vi "BACKUP_Keithley2450_and_24xx_plus_lockin_7_14_24.vi"() -> ()   [LabVIEW 2024]
uses:
  <vilib>/Analysis/1siggen.llb/Ramp Pattern by Delta.vi
  <vilib>/Utility/file.llb/Write Delimited Spreadsheet (string).vi
  <vilib>/Utility/file.llb/Write Delimited Spreadsheet (DBL).vi
  C:/Users/Public/OneDrive/Desktop/Keithley_2450_2470_1_4_0_LV2015_NewReadme2_2450-LV2015-1.4.0/Keithley 2450/Keithley 2450.lvlib
  <vilib>/Analysis/NI_AALBase.lvlib
  archive/Keithley 24XX/Keithley 24XX.lvlib
panel:
  out "XY Graph 3":cluster{dbl[], dbl[]}(graph)={[0.0, 0.05, 0.1, 0.15000000000000002, 0.2, 0.25, 0.30000000000000004, 0.35000000000000003, 0.4], [2.058748289029846, 2.0549935802361086, 2.025945473215966, 1.958083977655374, 1.8694392276726999, 1.770704656221769, 1.6639789912388152, 1.559635375168859, 1.4675568762085736]}
  out "current E field":dbl=0.4
  in  "d_t":dbl=17.0 format="%#_13g"
  in  "d_b":dbl=17.0 format="%#_13g"
  in  "E step":dbl=0.05 format="%#_13g"
  in  "E end":dbl=0.4 format="%#_13g"
  in  "E start (v/nm)":dbl format="%#_13g"
  out "current voltage 2450":dbl=6.7979141 format="%0.4f"
  in  "Reverse 2410":bool
  in  "Serial Configuration 2":T1={"Baud Rate"=9600, "Parity"=0, "Data Bits"=8, "Stop Bits"=10, "Flow Control"=0} {"Flow Control" items=["None", "XON/XOFF", "RTS/CTS", "XON/XOFF & RTS/CTS", "DTR/DSR", "XON/XOFF & DTR/DSR"]; "Stop Bits" items=["1.0"=10, "1.5"=15, "2.0"=20]; "Data Bits" items=["7"=7, "8"=8]; "Parity" items=["None", "Odd", "Even", "Mark", "Space"]; "Baud Rate" items=["300"=300, "600"=600, "1200"=1200, "2400"=2400, "4800"=4800, "9600"=9600, "19200"=19200]}
  in  "reset":bool
  in  "use 2540?":bool=TRUE
  out "XY Graph 2":cluster{dbl[], dbl[]}(graph)={[0.0, 0.05, 0.1, 0.15000000000000002, 0.2, 0.25, 0.30000000000000004, 0.35000000000000003, 0.4], [-0.0003388190682879211, 0.0003901722529266183, 1.3430241380812946e-05, 1.333691247717983e-05, 0.0001438023883998385, -0.0008806402301830829, -0.0010907914765878601, -0.0006143232866850923, -0.0016053824714035159]}
  out "XY Graph":cluster{dbl[], dbl[]}(graph)={[0.0, 0.05, 0.1, 0.15000000000000002, 0.2, 0.25, 0.30000000000000004, 0.35000000000000003, 0.4], [2.058748289029846, 2.0549935802361086, 2.025945473215966, 1.958083977655374, 1.8694392276726999, 1.770704656221769, 1.6639789912388152, 1.559635375168859, 1.4675568762085736]}
  in  "using 2400?":bool=TRUE
  out "current voltage 2410":dbl=-6.799285054206848 format="%0.4f"
  out "Current set voltage 2410":dbl=-6.800000000000001
  in  "V stepsize 2410":dbl
  in  "start V 2410":dbl
  in  "End V 2410":dbl
  out "standard deviation current measured 2450":dbl=1.0038305493714546e-08 format="%0.5e"
  out "mean current measured 2450":dbl=1.7421272433999997e-09 format="%0.5e"
  out "standard deviation current measured 2410":dbl=4.5644384533816545e-09 format="%0.5e"
  out "mean current measured 2410":dbl=-1.605382471403516e-09 format="%0.5e"
  in  "Compliance  Level 2410":dbl=5e-08
  in  "VISA resource name 2410":refnum<visa-resource-name>="GPIB0::16::INSTR"
  in  "Serial Configuration":T1={"Baud Rate"=9600, "Parity"=0, "Data Bits"=8, "Stop Bits"=10, "Flow Control"=0} {"Flow Control" items=["None", "XON/XOFF", "RTS/CTS", "XON/XOFF & RTS/CTS", "DTR/DSR", "XON/XOFF & DTR/DSR"]; "Stop Bits" items=["1.0"=10, "1.5"=15, "2.0"=20]; "Data Bits" items=["7"=7, "8"=8]; "Parity" items=["None", "Odd", "Even", "Mark", "Space"]; "Baud Rate" items=["300"=300, "600"=600, "1200"=1200, "2400"=2400, "4800"=4800, "9600"=9600, "19200"=19200]}
  in  "Wait for Current Meas":u32=100
  in  "Number of Current Meas":u32=20
  in  "Loop?":bool
  out "Current set voltage 2450":dbl=6.800000000000001
  in  "V stepsize 2450":dbl=0.5
  in  "start V 2450":dbl
  in  "End V 2450":dbl=2.0
  in  "Wait for lock in meas (ms)":i32=1000
  in  "File Path":path=path "C:/Users/Public/OneDrive/Desktop/test.txt"
  out "错误输出":errorcluster={"status"=FALSE, "code"=1073676294, "source"="VISA Read in OE1022D_Query_Data.vi->Keithley2450_and_24xx_plus_lockin_7_14_24.vi"}
  in  "Channel A Waveform Display":string(combo)="A-R"
  in  "Channel B Waveform Display":string(combo)="Channel_B_Rh1"
  out "AUX-ADC4 (V)":sgl format="%.3f"
  out "AUX-ADC3 (V)":sgl=0.0024414062 format="%.3f"
  out "AUX-ADC1 (V)":sgl format="%.3f"
  out "AUX-ADC2 (V)":sgl=0.0048828125 format="%.3f"
  out "R":sgl=0.0014845738 caption="R (Vrms)" format="%.3p"
  out "X":sgl=0.0014822832 caption="X (Vrms)" format="%.3p"
  out "Y":sgl=8.243722e-05 caption="Y (Vrms)" format="%.3p"
  out "θ (°)":sgl=3.183227 caption="θ (deg)" format="%.2f"
  out "频率 (Hz)":sgl=6040.048 caption="Freq (Hz)" format="%#.3f"
  out "噪声":sgl=1.6480133e-06 caption="Noise(Vrms)" format="%.3p"
  out "Rh1":sgl=9.916211e-05 caption="Rh1 (Vrms)" format="%.3p"
  out "θh1 (°)":sgl=90.1837 caption="θh1 (deg)" format="%.2f"
  out "Xh1":sgl=-3.1792828e-07 caption="Xh1 (Vrms)" format="%.3p"
  out "Yh1":sgl=9.91616e-05 caption="Yh1 (Vrms)" format="%.3p"
  out "X 2":sgl=4.511473e-07 caption="X (Vrms)" format="%.3p"
  out "Y 2":sgl=-4.716565e-07 caption="Y (Vrms)" format="%.3p"
  out "R 2":sgl=6.5268193e-07 caption="R (Vrms)" format="%.3p"
  out "θ (°) 2":sgl=-46.273182 caption="θ (deg)" format="%.2f"
  out "频率 (Hz) 2":sgl=50065.285 caption="Freq (Hz)" format="%#.3f"
  out "噪声 2":sgl=7.305374e-08 caption="Noise(Vrms)" format="%.3p"
  out "Xh1 2":sgl=1.594661e-05 caption="Xh1 (Vrms)" format="%.3p"
  out "Yh1 2":sgl=1.481611e-05 caption="Yh1 (Vrms)" format="%.3p"
  out "Rh1 2":sgl=2.1767211e-05 caption="Rh1 (Vrms)" format="%.3p"
  out "θh1 (°) 2":sgl=42.895382 caption="θh1 (deg)" format="%.2f"
  in  "A Sensitivity":u16(ring)=22 items=["1 nV/fA", "2 nV/fA", "5 nV/fA", "10 nV/fA", "20 nV/fA", "50 nV/fA", "100 nV/fA", "200 nV/fA", "500 nV/fA", "1 uV/pA", "2 uV/pA", "5 uV/pA", "10 uV/pA", "20 uV/pA", "50 uV/pA", "100 uV/pA", "200 uV/pA", "500 uV/pA", "1 mV/nA", "2 mV/nA", "5 mV/nA", "10 mV/nA", "20 mV/nA", "50 mV/nA", "100 mV/nA", "200 mV/nA", "500 mV/nA", "1 V/uA"]
  in  "B Sensitivity":u16(ring)=18 items=["1 nV/fA", "2 nV/fA", "5 nV/fA", "10 nV/fA", "20 nV/fA", "50 nV/fA", "100 nV/fA", "200 nV/fA", "500 nV/fA", "1 uV/pA", "2 uV/pA", "5 uV/pA", "10 uV/pA", "20 uV/pA", "50 uV/pA", "100 uV/pA", "200 uV/pA", "500 uV/pA", "1 mV/nA", "2 mV/nA", "5 mV/nA", "10 mV/nA", "20 mV/nA", "50 mV/nA", "100 mV/nA", "200 mV/nA", "500 mV/nA", "1 V/uA"]
  out "序列号":string="SSI LIA-OE1022D,SN:D6712164,Ver6.3200831"
  in  "Num Lock in Points":i32=100
  in  "OE1022D":refnum<visa-resource-name>="COM4"
  in  "Current Compliance Limit (0.1) 2450":dbl=5e-08
  in  "VISA resource name 2450":refnum<visa-resource-name>="GPIB0::1::INSTR"
  # "D:\\LabData\\XiaoWang_Group_data_2024on\\StackingTransitions\\CrI3\\dual_gate_round4\\d3\\RMCD\\Esweeps_0T_after_m2T\\stacked_location1_scan1.txt"
  # "C:\\Users\\Public\\OneDrive\\Desktop\\test.txt"
  # "instruments need to be reset before this runs. Run the sub vis that reset them. This has to be done because we do not reset in our program. That would turn off the output but we want to leave that on."
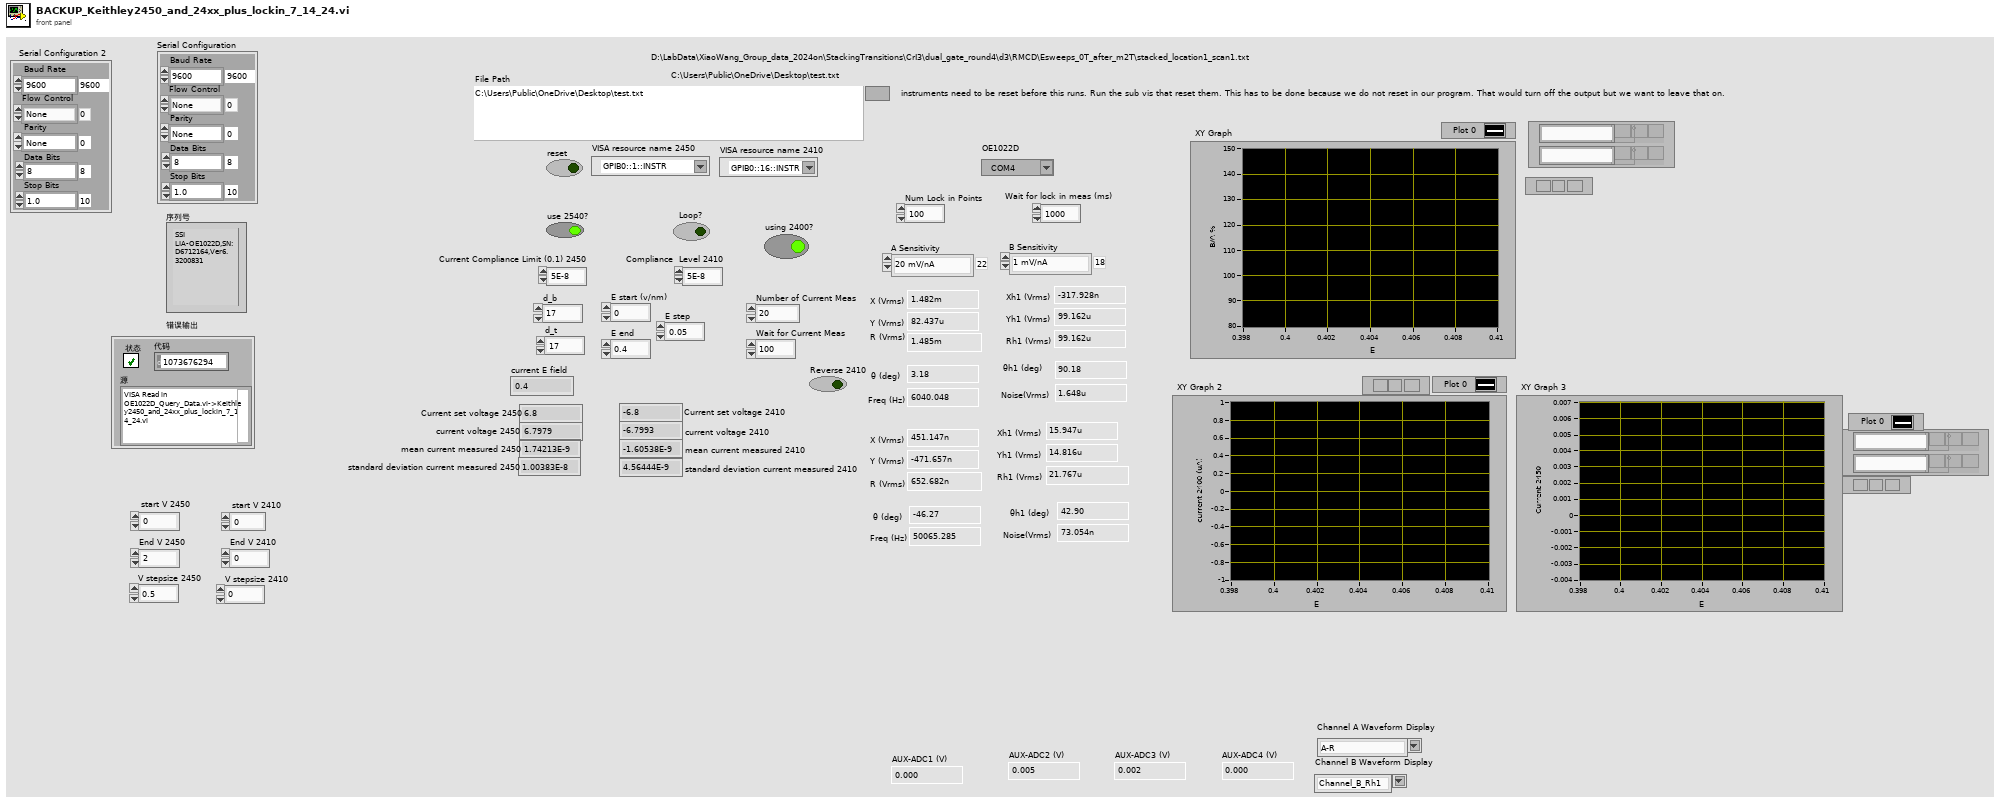
[diagram p1: front panel]
types:
  T1 = cluster{"Baud Rate":u32, "Parity":u16, "Data Bits":u16, "Stop Bits":u16, "Flow Control":u16}
  T2 = cluster{"AD1":dbl[], "AD2":dbl[], "AD3":dbl[], "AD4":dbl[]}
  T3 = cluster{"XB":dbl[], "YB":dbl[], "FrequencyB":dbl[], "NoiseB":dbl[], "Xh1B":dbl[], "Yh1B":dbl[], "Xh2B":dbl[], "Yh2B":dbl[], "Xh2B":dbl[]}
  T4 = cluster{"XA":dbl[], "YA":dbl[], "FrequencyA":dbl[], "NoiseA":dbl[], "Xh1A":dbl[], "Yh1A":dbl[], "Xh2A":dbl[], "Yh2A":dbl[]}
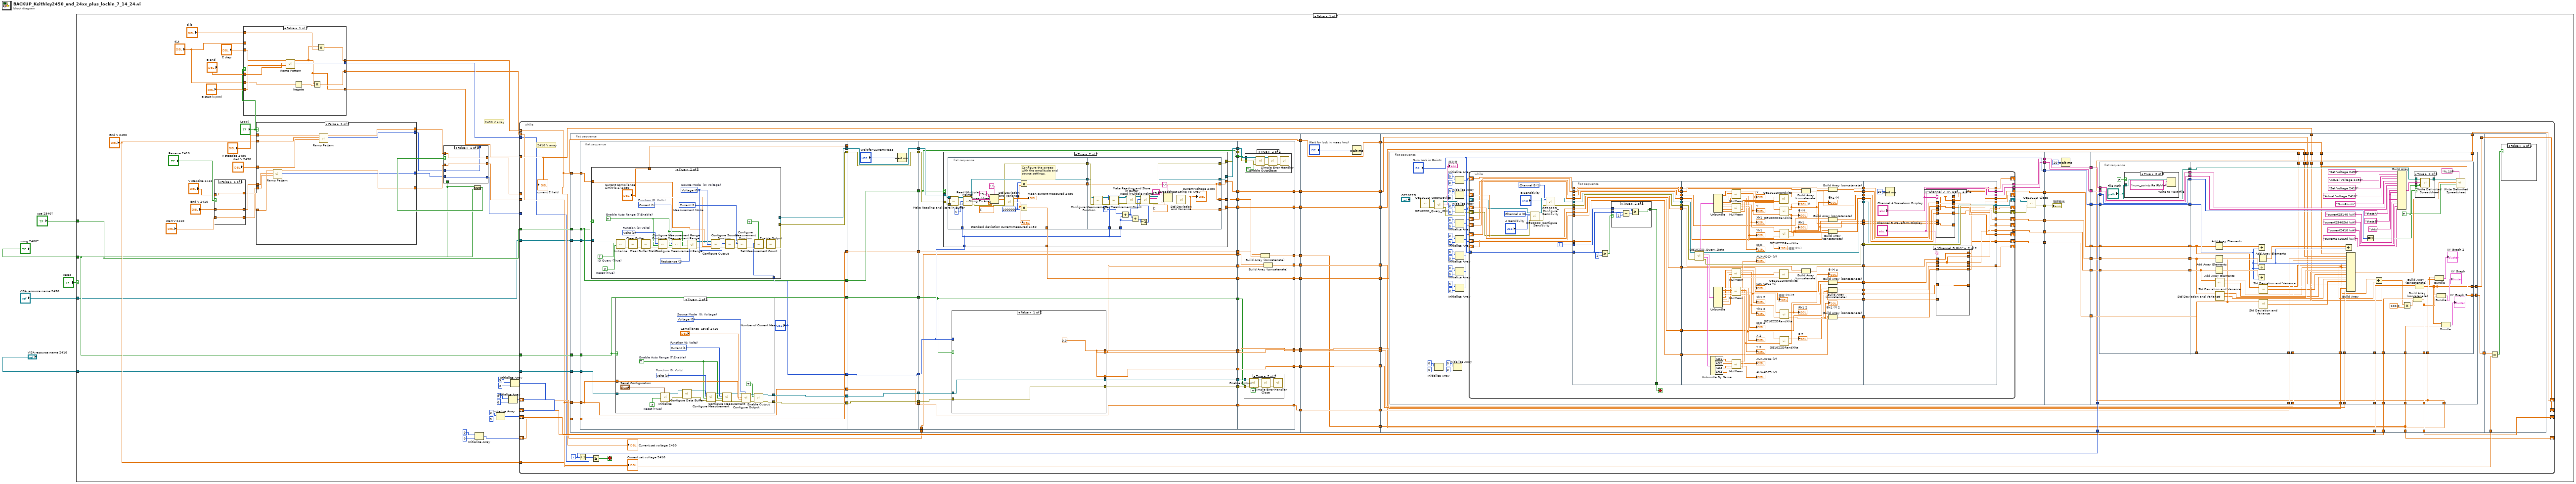
[diagram p0: block diagram]
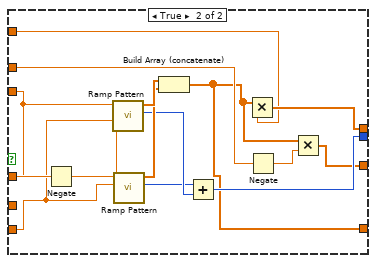
[diagram p2: hidden frame]
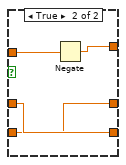
[diagram p3: hidden frame]
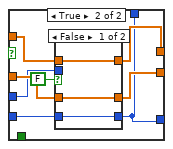
[diagram p4: hidden frame]
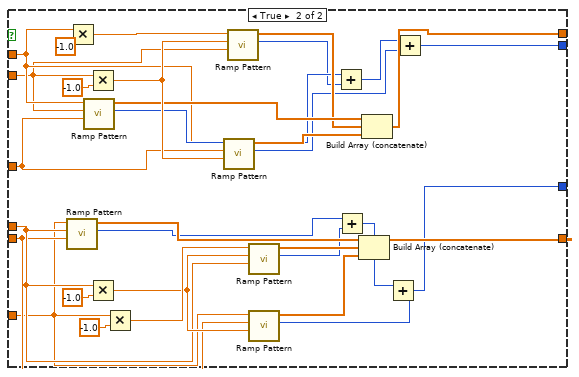
[diagram p6: hidden frame]
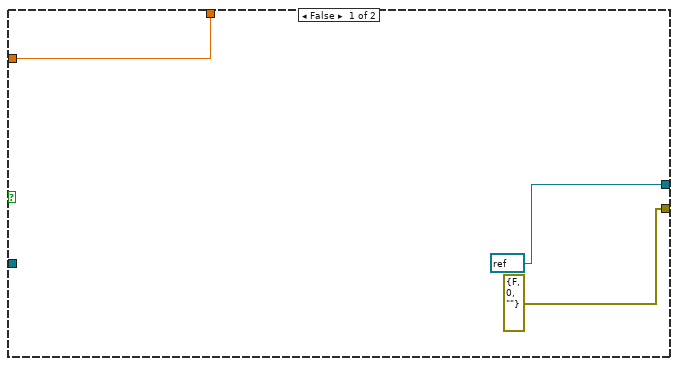
[diagram p7: hidden frame]
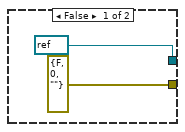
[diagram p8: hidden frame]
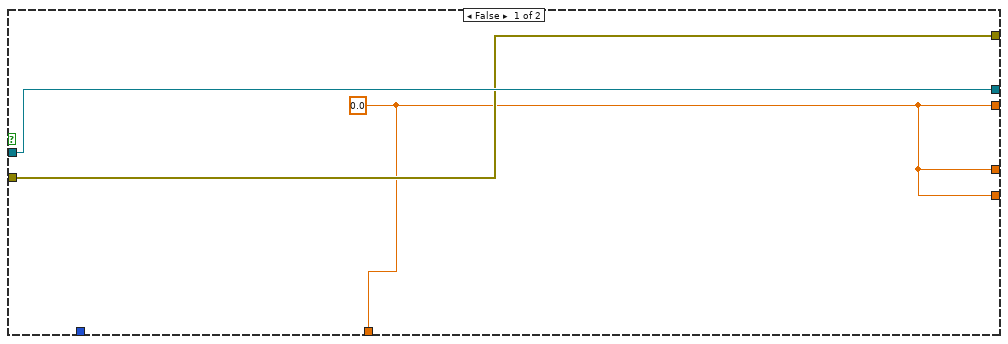
[diagram p9: hidden frame]
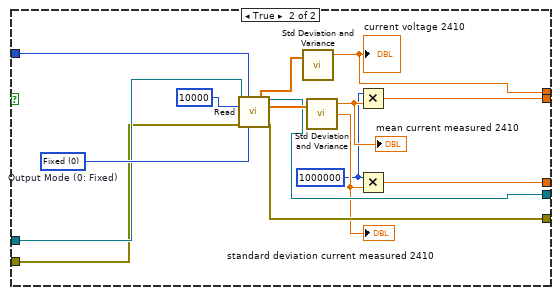
[diagram p10: hidden frame]
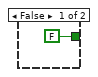
[diagram p13: hidden frame]
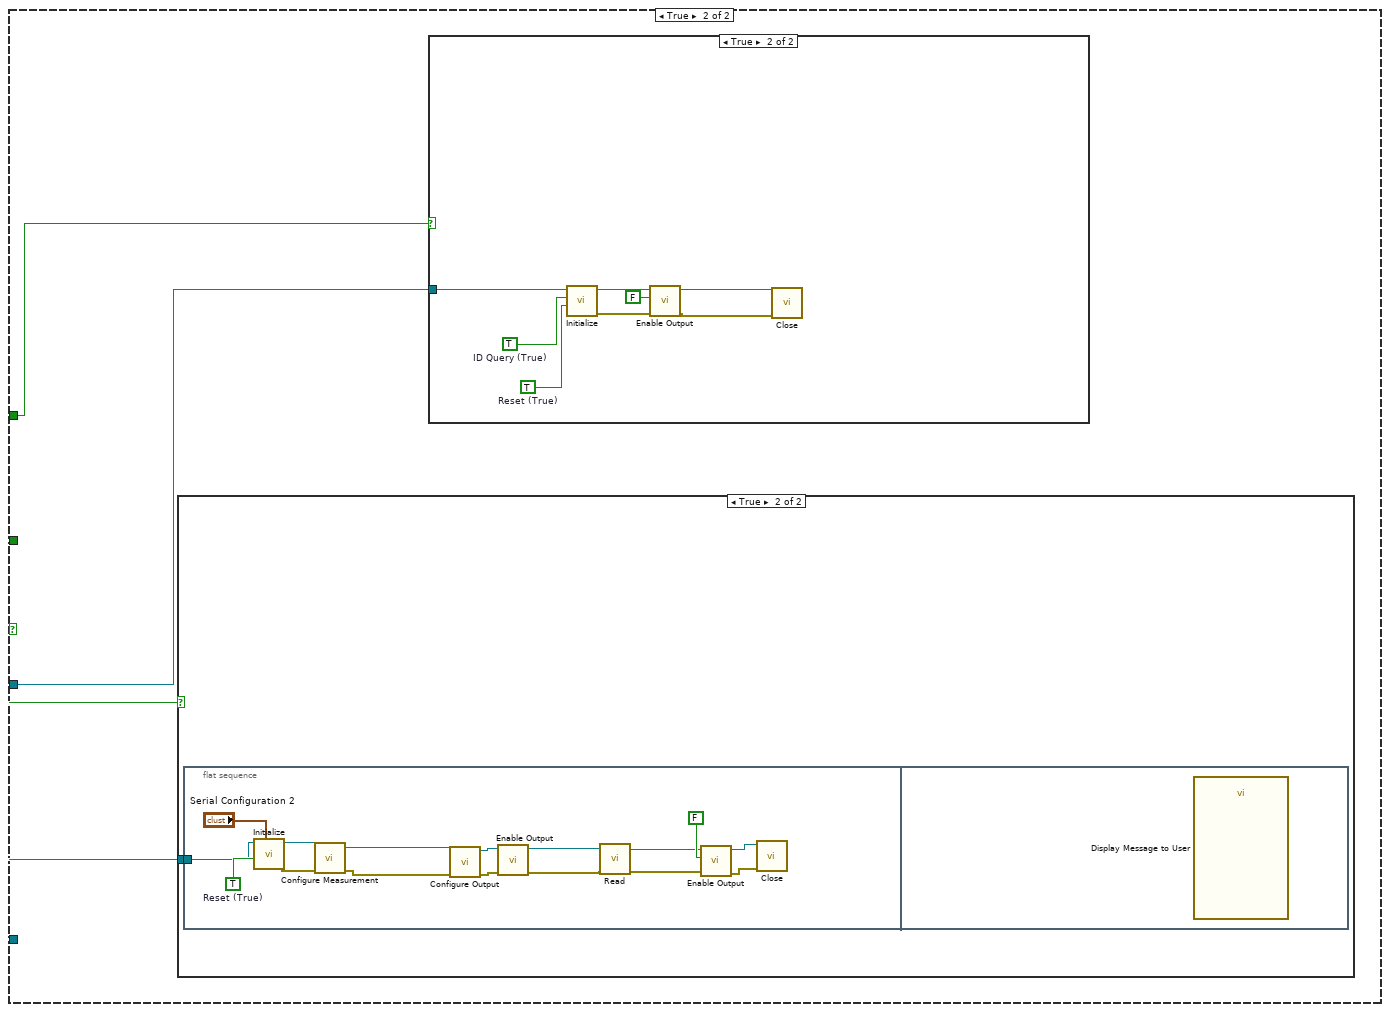
[diagram p19: hidden frame]
diagram:
  n1 = case shown="False" "reset" {
    tunnel: "using 2400?" -> [w32 w856]
    tunnel: "use 2540?" -> [w31 w857]
    tunnel: "VISA resource name 2410" -> [w30 w855]
    tunnel: "VISA resource name 2450" -> [w9 w854]
    frame False {
      # "2410 V array"
      # "2450 V array"
      n2 = case shown="False" "Reverse 2410" {
        tunnel: "End V 2410" -> [w77 w79]
        tunnel: [w77 w78] -> w27
        tunnel: "V stepsize 2410" -> [w76 w81]
        tunnel: [w76 w80] -> w25
        tunnel: "start V 2410" -> [w75 w78]
        tunnel: [w75 w79] -> w23
        frame False {
        }
        frame True {
          n3 = Negate(x=w81) -> (-x=w80:dbl)
        }
      }
      n4 = case shown="False" "Loop?" {
        tunnel: "E end" -> [w58 w74]
        tunnel: "E start (v/nm)" -> [w57 w73]
        tunnel: "E step" -> [w59 w72]
        tunnel: [w52 w65] -> w15
        tunnel: [w56 w66] -> w18
        tunnel: [w51 w64] -> w13
        tunnel: "d_b" -> [w53 w62]
        tunnel: "d_t" -> [_ w61]
        tunnel: "d_t" -> [w55 _]
        tunnel: [w50 w60] -> w14
        frame False {
          n5 = call-poly <vilib>:"Ramp Pattern.vi"("start"=w57, "end"=w58, "delta"=w59) -> ("samples"=w56:i32, "Ramp Pattern"=w50:dbl[])  [unwired: 6 in, 1 out]
          n6 = Negate(x=w55) -> (-x=w54:dbl)
          n7 = Multiply(x=w50, y=w54) -> (x*y=w51:dbl[])
          n8 = Multiply(x=w50, y=w53) -> (x*y=w52:dbl[])
        }
        frame True {
          n9 = Negate(x=w72) -> (-x=w71:dbl)
          n10 = call-poly <vilib>:"Ramp Pattern.vi"("start"=w73, "end"=w74, "delta"=w72) -> ("samples"=w68:i32, "Ramp Pattern"=w70:dbl[])  [unwired: 6 in, 1 out]
          n11 = call-poly <vilib>:"Ramp Pattern.vi"("start"=w74, "end"=w73, "delta"=w71) -> ("samples"=w67:i32, "Ramp Pattern"=w69:dbl[])  [unwired: 6 in, 1 out]
          n12 = Build Array (concatenate)(w70, w69) -> (w60:dbl[])
          n13 = Add(x=w67, y=w68) -> (x+y=w66:i32)
          n14 = Multiply(x=w60, y=w62) -> (x*y=w65:dbl[])
          n15 = Negate(x=w61) -> (-x=w63:dbl)
          n16 = Multiply(x=w60, y=w63) -> (x*y=w64:dbl[])
        }
      }
      n17 = case shown="False" "Loop?" {
        tunnel: [w105 w133] -> w36
        tunnel: [w104 w128] -> w34
        tunnel: "V stepsize 2450" -> [w106 w127]
        tunnel: "start V 2450" -> [w107 w126]
        tunnel: "End V 2450" -> [w108 w125]
        tunnel: w27 -> [w103 w113]
        tunnel: w25 -> [w101 w111]
        tunnel: w23 -> [w102 w112]
        tunnel: [w100 w110] -> w37
        tunnel: [w99 w109] -> w33
        frame False {
          n18 = call-poly <vilib>:"Ramp Pattern.vi"("start"=w102, "end"=w103, "delta"=w101) -> ("samples"=w99:i32, "Ramp Pattern"=w100:dbl[])  [unwired: 6 in, 1 out]
          n19 = call-poly <vilib>:"Ramp Pattern.vi"("start"=w107, "end"=w108, "delta"=w106) -> ("samples"=w104:i32, "Ramp Pattern"=w105:dbl[])  [unwired: 6 in, 1 out]
        }
        frame True {
          n20 = call-poly <vilib>:"Ramp Pattern.vi"("start"=w112, "end"=w113, "delta"=w111) -> ("samples"=w117:i32, "Ramp Pattern"=w120:dbl[])  [unwired: 6 in, 1 out]
          n21 = Multiply(x=w127, y=-1.0) -> (x*y=w138:dbl)
          n22 = call-poly <vilib>:"Ramp Pattern.vi"("start"=w126, "end"=w125, "delta"=w127) -> ("samples"=w132:i32, "Ramp Pattern"=w136:dbl[])  [unwired: 6 in, 1 out]
          n23 = Multiply(x=w125, y=-1.0) -> (x*y=w137:dbl)
          n24 = Multiply(x=w113, y=-1.0) -> (x*y=w121:dbl)
          n25 = Multiply(x=w111, y=-1.0) -> (x*y=w122:dbl)
          n26 = call-poly <vilib>:"Ramp Pattern.vi"("start"=w137, "end"=w126, "delta"=w127) -> ("samples"=w130:i32, "Ramp Pattern"=w134:dbl[])  [unwired: 6 in, 1 out]
          n27 = call-poly <vilib>:"Ramp Pattern.vi"("start"=w125, "end"=w137, "delta"=w138) -> ("samples"=w131:i32, "Ramp Pattern"=w135:dbl[])  [unwired: 6 in, 1 out]
          n28 = call-poly <vilib>:"Ramp Pattern.vi"("start"=w113, "end"=w121, "delta"=w122) -> ("samples"=w116:i32, "Ramp Pattern"=w119:dbl[])  [unwired: 6 in, 1 out]
          n29 = call-poly <vilib>:"Ramp Pattern.vi"("start"=w121, "end"=w112, "delta"=w111) -> ("samples"=w115:i32, "Ramp Pattern"=w118:dbl[])  [unwired: 6 in, 1 out]
          n30 = Add(x=w132, y=w131) -> (x+y=w129:i32)
          n31 = Add(x=w117, y=w116) -> (x+y=w114:i32)
          n32 = Build Array (concatenate)(w120, w119, w118) -> (w110:dbl[])
          n33 = Build Array (concatenate)(w136, w135, w134) -> (w133:dbl[])
          n34 = Add(x=w114, y=w115) -> (x+y=w109:i32)
          n35 = Add(x=w129, y=w130) -> (x+y=w128:i32)
        }
      }
      n36 = Exclusive Or(1:w32, 2:w31) -> (0:w35:bool)
      n37 = case shown="False" w35 {
        tunnel: w37 -> [w84 w93]
        tunnel: w36 -> [w85 w91]
        tunnel: [w85 w90] -> w11
        tunnel: [w84 w92] -> w12
        tunnel: w31 -> [_ _]
        tunnel: w34 -> [w83 w89]
        tunnel: w33 -> [w82 w88]
        tunnel: [w83 w86] -> _
        tunnel: [w82 w86] -> w10
        frame False {
        }
        frame True {
          n38 = case shown="False" FALSE {
            tunnel: w93 -> [w96 _]
            tunnel: [w96 w98] -> w92
            tunnel: w91 -> [w94 w98]
            tunnel: [w94 w98] -> w90
            tunnel: w89 -> [_ w97]
            tunnel: w88 -> [w95 _]
            tunnel: [w95 w97] -> w86
            frame False {
            }
            frame True {
            }
          }
        }
      }
      n39 = Initialize Array(0, 0) -> (w6:i32[])
      n40 = Initialize Array(0, 0) -> (w44:i32[])
      n41 = Initialize Array(0, 0) -> (w41:i32[])
      n42 = Initialize Array(0, 0) -> (w38:i32[])
      n43 = while {
        tunnel: w15 -> [w148] mode=indexing
        tunnel: w18 -> [w146]
        tunnel: "End V 2450" -> [w175]
        tunnel: w13 -> [w147] mode=indexing
        tunnel: w32 -> [w162]
        shift-right: [w160] -> _
        shift-left: w44 -> [w161]
        shift-right: [w159] -> _
        shift-left: w41 -> [w158]
        shift-right: [w154] -> _
        shift-left: w38 -> [w157]
        tunnel: w31 -> [w153]
        tunnel: w30 -> [w152]
        tunnel: w14 -> [w149] mode=indexing
        tunnel: w12 -> [_]
        tunnel: w11 -> [_]
        tunnel: w10 -> [_]
        tunnel: w9 -> [w145]
        shift-right: [w141] -> _
        shift-left: w6 -> [w144]
        i -> [w177]
        stop <- w181 stop-if-true
        n44 = flat-sequence {
          tunnel: w148 -> [w234]
          tunnel: [w234] -> w179
          tunnel: [w216] -> w173
          tunnel: [w215] -> w171
          tunnel: [w214] -> w169
          tunnel: [w213] -> w167
          tunnel: [w211] -> w165
          tunnel: [w207] -> w164
          tunnel: w147 -> [w206]
          tunnel: w162 -> [w203]
          tunnel: w157 -> [w198]
          tunnel: [w197] -> w155
          tunnel: w153 -> [w196]
          tunnel: w152 -> [w191]
          tunnel: [w189] -> w151
          tunnel: w145 -> [w188]
          tunnel: w144 -> [w186]
          tunnel: [w182] -> w142
          tunnel: w179 -> [w455]
          tunnel: [w455] -> w178
          tunnel: [w454] -> w174
          tunnel: w173 -> [w454]
          tunnel: [w453] -> w172
          tunnel: w171 -> [w453]
          tunnel: [w452] -> w170
          tunnel: w169 -> [w452]
          tunnel: [w451] -> w168
          tunnel: w167 -> [w451]
          tunnel: [w450] -> w166
          tunnel: w165 -> [w450]
          tunnel: w164 -> [w449]
          tunnel: [w449] -> w163
          tunnel: [w448] -> w156
          tunnel: w155 -> [w448]
          tunnel: w151 -> [w447]
          tunnel: [w447] -> w150
          tunnel: [w446] -> w143
          tunnel: w142 -> [w446]
          tunnel: w178 -> [w466]
          tunnel: w177 -> [w474]
          tunnel: [w473] -> w176
          tunnel: w174 -> [w468]
          tunnel: w172 -> [w467]
          tunnel: w170 -> [w472]
          tunnel: w168 -> [w471]
          tunnel: w166 -> [w470]
          tunnel: w163 -> [w469]
          tunnel: w161 -> [w465]
          tunnel: [w464] -> w160
          tunnel: [w463] -> w159
          tunnel: w158 -> [w462]
          tunnel: w156 -> [w461]
          tunnel: [w460] -> w154
          tunnel: w150 -> [w459]
          tunnel: w149 -> [w458]
          tunnel: w143 -> [w457]
          tunnel: [w457] -> w141
          tunnel: w176 -> [w852]
          tunnel: w175 -> [w853]
          frame #0 {
            n45 = flat-sequence {
              tunnel: w234 -> [w247]
              tunnel: [w239] -> w233
              tunnel: [w246] -> w231
              tunnel: [w240] -> w230
              tunnel: [w245] -> w228
              tunnel: [w244] -> w227
              tunnel: ["Number of Current Meas"] -> w221
              tunnel: [w243] -> w209
              tunnel: w206 -> [w243]
              tunnel: w203 -> [w242]
              tunnel: [w242] -> w201
              tunnel: w196 -> [w238]
              tunnel: [w238] -> w194
              tunnel: w191 -> [w237]
              tunnel: w188 -> [w236]
              tunnel: w186 -> [w235]
              tunnel: [w235] -> w183
              tunnel: w233 -> [w319]
              tunnel: [w319] -> w232
              tunnel: w231 -> [_]
              tunnel: w230 -> [w318]
              tunnel: [w318] -> w229
              tunnel: w228 -> [w316]
              tunnel: w227 -> [w315]
              tunnel: [w316] -> w226
              tunnel: [w315] -> w225
              tunnel: [w314] -> w222
              tunnel: w221 -> [w314]
              tunnel: [w313] -> w210
              tunnel: w209 -> [w313]
              tunnel: [w312] -> w202
              tunnel: w201 -> [w312]
              tunnel: [w311] -> w195
              tunnel: w194 -> [w311]
              tunnel: [w310] -> w184
              tunnel: w183 -> [w310]
              tunnel: w232 -> [w336]
              tunnel: w229 -> [w332]
              tunnel: w226 -> [w340]
              tunnel: w225 -> [w339]
              tunnel: [w338] -> w224
              tunnel: [w337] -> w223
              tunnel: w222 -> [w335]
              tunnel: [w334] -> w220
              tunnel: [w333] -> w219
              tunnel: [w328] -> w218
              tunnel: [w329] -> w217
              tunnel: [w330] -> w212
              tunnel: w210 -> [w331]
              tunnel: [w331] -> w208
              tunnel: [w324] -> w205
              tunnel: [w323] -> w204
              tunnel: w202 -> [w327]
              tunnel: [w327] -> w200
              tunnel: [w326] -> w199
              tunnel: w198 -> [w326]
              tunnel: w195 -> [w325]
              tunnel: [w325] -> w193
              tunnel: [w323] -> w192
              tunnel: [w322] -> w190
              tunnel: [w321] -> w187
              tunnel: [w320] -> w185
              tunnel: w184 -> [w320]
              tunnel: w224 -> [w433]
              tunnel: w223 -> [w432]
              tunnel: w220 -> [w431]
              tunnel: w219 -> [w430]
              tunnel: w218 -> [w423]
              tunnel: w217 -> [w429]
              tunnel: [w423] -> w216
              tunnel: [w429] -> w215
              tunnel: [w428] -> w214
              tunnel: [w427] -> w213
              tunnel: [w426] -> w211
              tunnel: w212 -> [w426]
              tunnel: w208 -> [w425]
              tunnel: [w425] -> w207
              tunnel: w205 -> [w427]
              tunnel: w204 -> [w428]
              tunnel: w200 -> [w424]
              tunnel: w199 -> [w422]
              tunnel: [w421] -> w197
              tunnel: w193 -> [w420]
              tunnel: w192 -> [w419]
              tunnel: w190 -> [w418]
              tunnel: [w418] -> w189
              tunnel: w187 -> [w417]
              tunnel: w185 -> [w416]
              tunnel: [w415] -> w182
              frame #0 {
                n46 = case shown="True" w238 {
                  tunnel: w247 -> [w250 w251]
                  tunnel: [w250 "Current Compliance Limit (0.1) 2450"] -> w246
                  tunnel: "Number of Current Meas" -> [_ w263]
                  tunnel: [errorcluster {"status"=FALSE, "code"=0, "source"=""} ("error out") w260] -> w240
                  tunnel: [refnum<visa-resource-name> refnum ("VISA resource name out") w259] -> w239
                  tunnel: w236 -> [_ w252]
                  frame False {
                  }
                  frame True {
                    w254 = u16 2 items=["Volts", "Current", "Resistance"] ("Function (0: Volts)")
                    w275 = u16 0 items=["Voltage", "Current"]  # Source Mode  (0: Voltage)
                    w276 = u16 1 items=["Volts", "Current", "Auto Resistance", "Manual Resistance", "Digitize Voltage", "Digitize Current"]  # Measurement Mode
                    w253 = TRUE  # Enable Auto Range (T:Enable)
                    w277 = u16 1 items=["Volts", "Current", "Resistance"]  # Function (0: Volts)
                    w278 = u16 0 items=["Volts", "Current", "Resistance"]  # Function (0: Volts)
                    w273 = FALSE  # Reset (True)
                    w279 = TRUE  # ID Query (True)
                    n47 = call "Initialize.vi"("Reset (True)"=w273, "ID Query (True)"=w279, "VISA resource name"=w252) -> ("error out"=w271:errorcluster, "VISA resource name out"=w272:refnum<visa-resource-name>)  [unwired: 7 in]
                    n48 = call "Clear Buffer.vi"("VISA resource name"=w272, "error in (no error)"=w271) -> ("VISA resource name out"=w270:refnum<visa-resource-name>, "error out"=w267:errorcluster)  [unwired: 12 in]
                    n49 = call "Clear Buffer Statistics.vi"("VISA resource name"=w270, "error in (no error)"=w267) -> ("VISA resource name out"=w269:refnum<visa-resource-name>, "error out"=w268:errorcluster)  [unwired: 12 in]
                    n50 = call "Configure Measurement Range.vi"("error in (no error)"=w268, "Enable Auto Range (T:Enable)"=w253, "Function (0: Volts)"=w278, "VISA resource name"=w269) -> ("error out"=w281:errorcluster, "VISA resource name out"=w280:refnum<visa-resource-name>)  [unwired: 6 in]
                    n51 = call "Configure Measurement Range.vi"("error in (no error)"=w281, "Enable Auto Range (T:Enable)"=w253, "Function (0: Volts)"=w277, "VISA resource name"=w280) -> ("error out"=w257:errorcluster, "VISA resource name out"=w258:refnum<visa-resource-name>)  [unwired: 6 in]
                    n52 = call "Configure Measurement Range.vi"("error in (no error)"=w257, "Enable Auto Range (T:Enable)"=w253, "Function (0: Volts)"=w254, "VISA resource name"=w258) -> ("error out"=w256:errorcluster, "VISA resource name out"=w255:refnum<visa-resource-name>)  [unwired: 6 in]
                    n53 = call "Configure Output.vi"("VISA resource name"=w255, "Source Level (0)"=w251, "Source Mode  (0: Voltage)"=w275, "Source Limit Level (0.1)"="Current Compliance Limit (0.1) 2450", "error in (no error)"=w256) -> ("VISA resource name out"=w282:refnum<visa-resource-name>, "error out"=w283:errorcluster)  [unwired: 9 in]
                    n54 = call "Configure Source Function.vi"("error in (no error)"=w283, "Function (0: Volts)"=w275, "VISA resource name"=w282) -> ("error out"=w284:errorcluster, "VISA resource name out"=w285:refnum<visa-resource-name>)  [unwired: 7 in]
                    n55 = call "Configure Measurement Function.vi"("error in (no error)"=w284, "Function (0: Volts)"=w276, "VISA resource name"=w285) -> ("error out"=w264:errorcluster, "VISA resource name out"=w262:refnum<visa-resource-name>)  [unwired: 7 in]
                    n56 = call "Set Measurement Count.vi"("error in (no error)"=w264, "Measurement Count"=w263, "VISA resource name"=w262) -> ("error out"=w265:errorcluster, "VISA resource name out"=w266:refnum<visa-resource-name>)  [unwired: 7 in]
                    n57 = call "Enable Output.vi"("error in (no error)"=w265, "Enable Output (T: Enable)"=TRUE, "VISA resource name"=w266) -> ("error out"=w260:errorcluster, "VISA resource name out"=w259:refnum<visa-resource-name>)  [unwired: 7 in]
                  }
                }
                n58 = case shown="True" w242 {
                  tunnel: [refnum<visa-resource-name> refnum ("VISA resource name out") w300] -> w245
                  tunnel: [errorcluster {"status"=FALSE, "code"=0, "source"=""} ("error out") w299] -> w244
                  tunnel: w243 -> [_ w297]
                  tunnel: w237 -> [_ w288]
                  frame False {
                  }
                  frame True {
                    w296 = FALSE  # Reset (True)
                    w298 = u16 0 items=["Voltage", "Current"]  # Source Mode  (0: Voltage)
                    w295 = TRUE  # Enable Auto Range (T:Enable)
                    w306 = u16 1 items=["Volts", "Current", "Resistance"]  # Function (0: Volts)
                    w305 = u16 0 items=["Volts", "Current", "Resistance"]  # Function (0: Volts)
                    n59 = call "Initialize.vi"("Serial Configuration"="Serial Configuration", "Reset (True)"=w296, "VISA resource name"=w288) -> ("error out"=w291:errorcluster, "VISA resource name out"=w292:refnum<visa-resource-name>)  [unwired: 7 in]
                    n60 = call "Configure Data Buffer.vi"("error in (no error)"=w291, "VISA resource name"=w292) -> ("error out"=w290:errorcluster, "VISA resource name out"=w289:refnum<visa-resource-name>)  [unwired: 8 in]
                    n61 = call "Configure Measurement.vi"("error in (no error)"=w290, "Enable Auto Range (T:Enable)"=w295, "Function (0: Volts)"=w305, "VISA resource name"=w289) -> ("error out"=w301:errorcluster, "VISA resource name out"=w302:refnum<visa-resource-name>)  [unwired: 6 in]
                    n62 = call "Configure Measurement.vi"("error in (no error)"=w301, "Enable Auto Range (T:Enable)"=w295, "Function (0: Volts)"=w306, "VISA resource name"=w302) -> ("error out"=w293:errorcluster, "VISA resource name out"=w294:refnum<visa-resource-name>)  [unwired: 6 in]
                    n63 = call "Configure Output.vi"("Source Mode  (0: Voltage)"=w298, "error in (no error)"=w293, "Compliance  Level (0.1)"="Compliance  Level 2410", "Output Level (0)"=w297, "VISA resource name"=w294) -> ("error out"=w309:errorcluster, "VISA resource name out"=w308:refnum<visa-resource-name>)  [unwired: 5 in]
                    n64 = call "Enable Output.vi"("error in (no error)"=w309, "Enable Output (T: Enable)"=TRUE, "VISA resource name"=w308) -> ("error out"=w299:errorcluster, "VISA resource name out"=w300:refnum<visa-resource-name>)  [unwired: 7 in]
                  }
                }
              }
              frame #1 {
                n65 = Wait (ms)(milliseconds to wait="Wait for Current Meas") -> ()  [unwired: 1 out]
              }
              frame #2 {
                n66 = case shown="True" w325 {
                  tunnel: w336 -> [w343 w355]
                  tunnel: w335 -> [_ w346]
                  tunnel: [w343 w354] -> w334
                  tunnel: [w342 w353] -> w333
                  tunnel: w332 -> [w342 w352]
                  tunnel: [w341 w351] -> w329
                  tunnel: [w341 w350] -> w328
                  tunnel: [w341 w345] -> w322
                  tunnel: [w341 w344] -> w321
                  frame False {
                    w341 = 0.0
                  }
                  frame True {
                    n67 = flat-sequence {
                      tunnel: w355 -> [w373]
                      tunnel: w346 -> [w370]
                      tunnel: w352 -> [w361]
                      tunnel: [w360] -> w351
                      tunnel: [w364] -> w349
                      tunnel: [w363] -> w348
                      tunnel: [w358] -> w347
                      tunnel: [w374] -> w350
                      tunnel: [w391] -> w353
                      tunnel: [w388] -> w354
                      tunnel: w349 -> [w389]
                      tunnel: w348 -> [w390]
                      tunnel: w347 -> [w374]
                      tunnel: w346 -> [w378]
                      tunnel: w346 -> [w376]
                      tunnel: [w375] -> w345
                      tunnel: [w374] -> w344
                      frame #0 {
                        w356 = 1000000 ("Timeout (10000 ms)")
                        # "Configure the sweep with the amplitude and source settings."
                        n68 = call "Make Reading and Store in Buffer.vi"("VISA resource name"=w373, "error in (no error)"=w361) -> ("VISA resource name out"=w371:refnum<visa-resource-name>, "error out"=w372:errorcluster)  [unwired: 12 in]
                        n69 = call "Read (Multiple Points).vi"("VISA resource name"=w371, "Start Index (1)"=u32 1, "End Index (1)"=w370, "error in (no error)"=w372) -> ("VISA resource name out"=w364:refnum<visa-resource-name>, "Data out"=w365:string, "error out"=w363:errorcluster)  [unwired: 9 in]
                        n70 = Spreadsheet String To Array(delimiter (Tab)=",", format string="%s", spreadsheet string=w365, array type (2D Dbl)=dbl[] []) -> (array=w362:dbl[])
                        n71 = call <vilib>:"Std Deviation and Variance.vi"("X"=w362) -> ("mean"=w357:dbl, "standard deviation"=w359:dbl)  [unwired: 1 in, 1 out]
                        "mean current measured 2450" <- w357
                        "standard deviation current measured 2450" <- w359
                        n72 = Multiply(x=w356, y=w357) -> (x*y=w358:dbl)
                        n73 = Multiply(x=w359, y=w356) -> (x*y=w360:dbl)
                      }
                      frame #1 {
                        n74 = call "Configure Measurement Function.vi"("error in (no error)"=w390, "VISA resource name"=w389) -> ("error out"=w392:errorcluster, "VISA resource name out"=w396:refnum<visa-resource-name>)  [unwired: 8 in]
                        n75 = call "Set Measurement Count.vi"("error in (no error)"=w392, "Measurement Count"=w376, "VISA resource name"=w396) -> ("error out"=w393:errorcluster, "VISA resource name out"=w387:refnum<visa-resource-name>)  [unwired: 7 in]
                        n76 = Add(x=u32 1 ("Start Index (1)"), y=w378) -> (x+y=w379:u32)
                        n77 = call "Make Reading and Store in Buffer.vi"("VISA resource name"=w387, "error in (no error)"=w393) -> ("VISA resource name out"=w395:refnum<visa-resource-name>, "error out"=w394:errorcluster)  [unwired: 12 in]
                        n78 = Add(x=w379, y=w378) -> (x+y=w380:u32)
                        n79 = Decrement(x=w380) -> (x-1=w377:u32)
                        n80 = call "Read (Multiple Points).vi"("VISA resource name"=w395, "Start Index (1)"=w379, "End Index (1)"=w377, "error in (no error)"=w394) -> ("VISA resource name out"=w388:refnum<visa-resource-name>, "Data out"=w383:string, "error out"=w391:errorcluster)  [unwired: 9 in]
                        n81 = Spreadsheet String To Array(delimiter (Tab)=",", format string="%s", spreadsheet string=w383, array type (2D Dbl)=dbl[] []) -> (array=w382:dbl[])
                        n82 = call <vilib>:"Std Deviation and Variance.vi"("X"=w382) -> ("mean"=w375:dbl)  [unwired: 1 in, 2 out]
                        "current voltage 2450" <- w375
                      }
                    }
                  }
                }
                n83 = case shown="False" w327 {
                  tunnel: w340 -> [w399 w411]
                  tunnel: w339 -> [w398 w410]
                  tunnel: [w398 w409] -> w338
                  tunnel: [w399 w408] -> w337
                  tunnel: w335 -> [_ w407]
                  tunnel: [w397 w405] -> w330
                  tunnel: [w397 w404] -> w324
                  tunnel: [w397 w401] -> w323
                  frame False {
                    w397 = 0.0 ("mean")
                  }
                  frame True {
                    w400 = 1000000 ("Timeout (10000 ms)")
                    w413 = u16 0 items=["Fixed", "Sweep", "List"]  # Output Mode (0: Fixed)
                    n84 = call-poly "Read.vi"("VISA resource name"=w411, "Sample Count (1)"=w407, "Timeout (10000 ms)"=10000, "error in (no error)"=w410, "Output Mode (0: Fixed)"=w413) -> ("Voltage"=w406:sgl[], "VISA resource name out"=w408:refnum<visa-resource-name>, "Current"=w412:sgl[], "error out"=w409:errorcluster)  [unwired: 4 in, 3 out]
                    n85 = call <vilib>:"Std Deviation and Variance.vi"("X"=w406) -> ("mean"=w405:dbl)  [unwired: 1 in, 2 out]
                    "current voltage 2410" <- w405
                    n86 = call <vilib>:"Std Deviation and Variance.vi"("X"=w412) -> ("mean"=w402:dbl, "standard deviation"=w403:dbl)  [unwired: 1 in, 1 out]
                    "mean current measured 2410" <- w402
                    "standard deviation current measured 2410" <- w403
                    n87 = Multiply(x=w400, y=w402) -> (x*y=w401:dbl)
                    n88 = Multiply(x=w400, y=w403) -> (x*y=w404:dbl)
                  }
                }
              }
              frame #3 {
                n89 = case shown="True" w424 {
                  tunnel: w433 -> [_ w445]
                  tunnel: w432 -> [_ w444]
                  frame False {
                  }
                  frame True {
                    n90 = call "Enable Output.vi"("error in (no error)"=w445, "Enable Output (T: Enable)"=TRUE, "VISA resource name"=w444) -> ("error out"=w442:errorcluster, "VISA resource name out"=w443:refnum<visa-resource-name>)  [unwired: 7 in]
                    n91 = call "Close.vi"("error in (no error)"=w442, "VISA resource name"=w443) -> ("error out"=w441:errorcluster)  [unwired: 9 in]
                    n92 = call <vilib>:"Simple Error Handler.vi"("error in (no error)"=w441) -> ()  [unwired: 4 in, 5 out]
                  }
                }
                n93 = case shown="True" w420 {
                  tunnel: w431 -> [_ w439]
                  tunnel: w430 -> [_ w438]
                  frame False {
                  }
                  frame True {
                    n94 = call "Enable Output.vi"("error in (no error)"=w438, "Enable Output (T: Enable)"=TRUE, "VISA resource name"=w439) -> ("error out"=w435:errorcluster, "VISA resource name out"=w436:refnum<visa-resource-name>)  [unwired: 7 in]
                    n95 = call "Close.vi"("error in (no error)"=w435, "VISA resource name"=w436) -> ("error out"=w434:errorcluster)  [unwired: 9 in]
                    n96 = call <vilib>:"Simple Error Handler.vi"("error in (no error)"=w434) -> ()  [unwired: 4 in, 5 out]
                  }
                }
                n97 = Build Array (concatenate)(w416, w417) -> (w415:dbl[])
                n98 = Build Array (concatenate)(w422, w419) -> (w421:dbl[])
              }
            }
          }
          frame #1 {
            n99 = Wait (ms)(milliseconds to wait="Wait for lock in meas (ms)") -> ()  [unwired: 1 out]
          }
          frame #2 {
            n100 = flat-sequence {
              tunnel: [w510] -> w489
              tunnel: [w509] -> w488
              tunnel: ["Num Lock in Points"] -> w487
              tunnel: [w504] -> w486
              tunnel: [w508] -> w485
              tunnel: [w507] -> w484
              tunnel: [w494] -> w483
              tunnel: [w495] -> w482
              tunnel: w489 -> [w742]
              tunnel: [w742] -> w481
              tunnel: w488 -> [w741]
              tunnel: [w741] -> w480
              tunnel: w487 -> [w740]
              tunnel: [w740] -> w479
              tunnel: w486 -> [w738]
              tunnel: [w737] -> w478
              tunnel: w485 -> [w737]
              tunnel: w484 -> [w736]
              tunnel: [w736] -> w477
              tunnel: [w735] -> w476
              tunnel: w483 -> [w735]
              tunnel: w482 -> [w734]
              tunnel: [w734] -> w475
              tunnel: w481 -> [w770]
              tunnel: w480 -> [w769]
              tunnel: w479 -> [w768]
              tunnel: w478 -> [w766]
              tunnel: w477 -> [w765]
              tunnel: w476 -> [w763]
              tunnel: w475 -> [w761]
              tunnel: w474 -> [w759]
              tunnel: [w758] -> w473
              tunnel: w472 -> [w757]
              tunnel: w471 -> [w756]
              tunnel: w470 -> [w754]
              tunnel: w469 -> [w755]
              tunnel: w468 -> [w753]
              tunnel: w467 -> [w752]
              tunnel: w466 -> [w751]
              tunnel: w465 -> [w750]
              tunnel: [w749] -> w464
              tunnel: [w748] -> w463
              tunnel: w462 -> [w747]
              tunnel: w461 -> [w746]
              tunnel: [w746] -> w460
              tunnel: w459 -> [w745]
              tunnel: w458 -> [w744]
              tunnel: w457 -> [w743]
              frame #0 {
                n101 = call "OE1022D_OpenDevice.vi"("VISA resource name"="OE1022D") -> ("VISA资源名称输出"=w532:refnum<visa-resource-name>, "错误输出"=w531:errorcluster)  [unwired: 17 in]
                n102 = call "OE1022D_Query_IDN.vi"("错误输入（无错误）"=w531, "VISA resource name"=w532) -> ("错误输出"=w502:errorcluster, "序列号"=→"序列号":string, "VISA resource name out"=w503:refnum<visa-resource-name>)  [unwired: 1 in]
                n103 = Initialize Array(0, 0) -> ()  [unwired: 1 out]
                n104 = Initialize Array(0, 0) -> ()  [unwired: 1 out]
                n105 = Initialize Array(0, 0) -> (w528:i32[])
                n106 = Initialize Array(0, 0) -> (w512:i32[])
                n107 = Initialize Array(0, 0) -> (w511:i32[])
                n108 = Initialize Array(0, 0) -> (w497:i32[])
                n109 = Initialize Array(0, 0) -> (w517:i32[])
                n110 = Initialize Array(0, 0) -> (w518:i32[])
                n111 = Initialize Array(0, 0) -> (w496:i32[])
                n112 = Initialize Array(0, 0) -> (w523:i32[])
                n113 = while {
                  shift-right: [w589] -> _
                  shift-left: w528 -> [w588]
                  shift-right: [w586] -> _
                  shift-left: w523 -> [w585]
                  tunnel: "Num Lock in Points" -> [w578]
                  shift-right: [w566] -> _
                  shift-left: w517 -> [w568]
                  shift-right: [w562] -> _
                  shift-left: w518 -> [w565]
                  shift-right: [w555] -> _
                  shift-left: w511 -> [w561]
                  shift-right: [w554] -> _
                  shift-left: w512 -> [w560]
                  tunnel: [w553] -> w510
                  tunnel: [w552] -> w509
                  tunnel: [w551] -> w508
                  tunnel: [w550] -> w507
                  shift-right: [w549] -> w506
                  shift-left: w502 -> [w546]
                  shift-right: [w548] -> w505
                  shift-left: w503 -> [w547]
                  shift-right: [w538] -> w494
                  shift-left: w497 -> [w542]
                  shift-right: [w539] -> w495
                  shift-left: w496 -> [w540]
                  i -> [w580]
                  stop <- w579 stop-if-true
                  w571 = u8 1 items=["Channel A", "Channel B"] ("OE1022D A/B")
                  w577 = u8 0 items=["Channel A", "Channel B"] ("OE1022D A/B")
                  n114 = call "OE1022D_Configure Sensitivity.vi"("VISA resource name"=w547, "OE1022D A/B"=w577, "Sensitivity"="A Sensitivity", "error in (no error)"=w546) -> ("VISA resource name out"=w572:refnum<visa-resource-name>, "error out"=w573:errorcluster)  [unwired: 14 in]
                  n115 = call "OE1022D_Configure Sensitivity.vi"("VISA resource name"=w572, "OE1022D A/B"=w571, "Sensitivity"="B Sensitivity", "error in (no error)"=w573) -> ("VISA resource name out"=w575:refnum<visa-resource-name>, "error out"=w574:errorcluster)  [unwired: 14 in]
                  n116 = flat-sequence {
                    tunnel: w585 -> [w604]
                    tunnel: w588 -> [w605]
                    tunnel: w575 -> [w606]
                    tunnel: w574 -> [w607]
                    tunnel: [w607] -> w584
                    tunnel: [w606] -> w583
                    tunnel: [w605] -> w582
                    tunnel: [w604] -> w581
                    tunnel: w580 -> [w603]
                    tunnel: [w602] -> w579
                    tunnel: w578 -> [w600]
                    tunnel: [w598] -> w569
                    tunnel: w568 -> [w598]
                    tunnel: w565 -> [w597]
                    tunnel: [w597] -> w564
                    tunnel: w561 -> [w596]
                    tunnel: w560 -> [w595]
                    tunnel: [w596] -> w559
                    tunnel: [w595] -> w558
                    tunnel: [w594] -> w543
                    tunnel: w542 -> [w594]
                    tunnel: [w593] -> w541
                    tunnel: w540 -> [w593]
                    tunnel: [w684] -> w592
                    tunnel: [w683] -> w591
                    tunnel: [w637] -> w590
                    tunnel: [w634] -> w587
                    tunnel: w584 -> [w686]
                    tunnel: w583 -> [w685]
                    tunnel: w582 -> [w638]
                    tunnel: w581 -> [w636]
                    tunnel: w569 -> [w633]
                    tunnel: [w632] -> w567
                    tunnel: w564 -> [w630]
                    tunnel: [w629] -> w563
                    tunnel: w559 -> [w626]
                    tunnel: w558 -> [w627]
                    tunnel: [w625] -> w557
                    tunnel: [w624] -> w556
                    tunnel: [w620] -> w545
                    tunnel: [w622] -> w544
                    tunnel: w543 -> [w619]
                    tunnel: w541 -> [w618]
                    tunnel: [w617] -> w537
                    tunnel: [w616] -> w536
                    tunnel: [w615] -> w535
                    tunnel: [w614] -> w534
                    tunnel: w592 -> [w711]
                    tunnel: w591 -> [w712]
                    tunnel: w590 -> [w710]
                    tunnel: [w708] -> w589
                    tunnel: w587 -> [w704]
                    tunnel: [w703] -> w586
                    tunnel: [w712] -> w548
                    tunnel: [w711] -> w549
                    tunnel: w567 -> [w709]
                    tunnel: [w707] -> w566
                    tunnel: w563 -> [w706]
                    tunnel: [w705] -> w562
                    tunnel: w557 -> [w699]
                    tunnel: w556 -> [w702]
                    tunnel: [w701] -> w555
                    tunnel: [w700] -> w554
                    tunnel: [w698] -> w553
                    tunnel: [w697] -> w552
                    tunnel: ["Channel A Waveform Display"] -> w551
                    tunnel: ["Channel B Waveform Display"] -> w550
                    tunnel: w545 -> [w693]
                    tunnel: [w692] -> w538
                    tunnel: [w691] -> w539
                    tunnel: w544 -> [w694]
                    tunnel: w537 -> [w690]
                    tunnel: w536 -> [w689]
                    tunnel: w535 -> [w688]
                    tunnel: w534 -> [w687]
                    frame #0 {
                      n117 = Greater Or Equal?(x=w600, y=1) -> (x >= y?=w599:bool)
                      n118 = case shown="True" w599 {
                        tunnel: w603 -> [_ w613]
                        tunnel: [FALSE w612] -> w602
                        tunnel: w600 -> [_ w609]
                        frame False {
                        }
                        frame True {
                          n119 = Subtract(x=w609, y=1) -> (x-y=w610:i32)
                          n120 = Greater Or Equal?(x=w613, y=w610) -> (x >= y?=w612:bool)
                        }
                      }
                    }
                    frame #1 {
                      n121 = call "OE1022D_Query_Data.vi"("错误输入（无错误）"=w686, "VISA resource name"=w685) -> ("error out"=w684:errorcluster, "输出簇ADC"=w640:T2, "输出簇B"=w639:T3, "VISA resource name out"=w683:refnum<visa-resource-name>, "输出簇A"=w635:T4)  [unwired: 3 in]
                      n122 = Unbundle By Name(w640) -> ("AD1"=w679:dbl[], "AD2"=w680:dbl[], "AD3"=w681:dbl[], "AD4"=w682:dbl[])
                      n123 = Unbundle(w635) -> ("XA"=w645:dbl[], "YA"=w646:dbl[], "FrequencyA"=w647:dbl[], "NoiseA"=w648:dbl[], "Xh1A"=w653:dbl[], "Yh1A"=w654:dbl[], "Xh2A"=w655:dbl[], "Yh2A"=w656:dbl[])
                      n124 = Unbundle(w639) -> ("XB"=w669:dbl[], "YB"=w668:dbl[], "FrequencyB"=w667:dbl[], "NoiseB"=w666:dbl[], "Xh1B"=w665:dbl[], "Yh1B"=w664:dbl[], "Xh2B"=w663:dbl[], "Yh2B"=w662:dbl[])  [unwired: 1 out]
                      n125 = call "MulMean.vi"("IN 4"=w648, "IN 3"=w647, "IN 2"=w646, "IN 1"=w645) -> ("mean 4"=→"噪声":dbl, "mean 3"=→"频率 (Hz)":dbl, "mean 2"=w651:dbl, "mean 1"=w650:dbl)  [unwired: 4 in]
                      "X" <- w650
                      "Y" <- w651
                      n126 = call "MulMean.vi"("IN 4"=w656, "IN 3"=w655, "IN 2"=w654, "IN 1"=w653) -> ("mean 4"=w661:dbl, "mean 3"=w660:dbl, "mean 2"=w658:dbl, "mean 1"=w657:dbl)  [unwired: 4 in]
                      "Xh1" <- w657
                      "Yh1" <- w658
                      n127 = call "MulMean.vi"("IN 4"=w662, "IN 3"=w663, "IN 2"=w664, "IN 1"=w665) -> ("mean 4"=w678:dbl, "mean 3"=w677:dbl, "mean 2"=w676:dbl, "mean 1"=w675:dbl)  [unwired: 4 in]
                      "Xh1 2" <- w675
                      "Yh1 2" <- w676
                      n128 = call "MulMean.vi"("IN 4"=w666, "IN 3"=w667, "IN 2"=w668, "IN 1"=w669) -> ("mean 4"=→"噪声 2":dbl, "mean 3"=→"频率 (Hz) 2":dbl, "mean 2"=w674:dbl, "mean 1"=w673:dbl)  [unwired: 4 in]
                      "X 2" <- w673
                      "Y 2" <- w674
                      n129 = call "MulMean.vi"("IN 4"=w682, "IN 3"=w681, "IN 2"=w680, "IN 1"=w679) -> ("mean 4"=→"AUX-ADC4 (V)":dbl, "mean 3"=→"AUX-ADC3 (V)":dbl, "mean 2"=→"AUX-ADC2 (V)":dbl, "mean 1"=→"AUX-ADC1 (V)":dbl)  [unwired: 4 in]
                      n130 = call "OE1022DRandXita.vi"("Y"=w661, "X"=w660) -> ("R"=w631:dbl)  [unwired: 1 out]
                      n131 = call "OE1022DRandXita.vi"("Y"=w678, "X"=w677) -> ("R"=w628:dbl)  [unwired: 1 out]
                      n132 = call "OE1022DRandXita.vi"("Y"=w658, "X"=w657) -> ("θ (°)"=→"θh1 (°)":dbl, "R"=w614:dbl)
                      "Rh1" <- w614
                      n133 = call "OE1022DRandXita.vi"("Y"=w676, "X"=w675) -> ("θ (°)"=w623:dbl, "R"=w617:dbl)
                      "Rh1 2" <- w617
                      "θh1 (°) 2" <- w623
                      n134 = call "OE1022DRandXita.vi"("Y"=w674, "X"=w673) -> ("θ (°)"=→"θ (°) 2":dbl, "R"=w616:dbl)
                      "R 2" <- w616
                      n135 = call "OE1022DRandXita.vi"("Y"=w651, "X"=w650) -> ("θ (°)"=w621:dbl, "R"=w615:dbl)
                      "R" <- w615
                      "θ (°)" <- w621
                      n136 = Build Array (concatenate)(w630, w631) -> (w629:dbl[])
                      n137 = Build Array (concatenate)(w627, w628) -> (w624:dbl[])
                      n138 = Build Array (concatenate)(w638, w615) -> (w637:dbl[])
                      n139 = Build Array (concatenate)(w633, w614) -> (w632:dbl[])
                      n140 = Build Array (concatenate)(w619, w621) -> (w620:dbl[])
                      n141 = Build Array (concatenate)(w626, w617) -> (w625:dbl[])
                      n142 = Build Array (concatenate)(w636, w616) -> (w634:dbl[])
                      n143 = Build Array (concatenate)(w618, w623) -> (w622:dbl[])
                    }
                    frame #2 {
                      n144 = Wait (ms)(milliseconds to wait=10) -> ()  [unwired: 1 out]
                      n145 = case shown="\"Channel_A_R\", Default" "Channel A Waveform Display" {
                        tunnel: w710 -> [w728 w731]
                        tunnel: [w728 w731] -> w708
                        tunnel: w709 -> [w726 w733]
                        tunnel: [w726 w733] -> w707
                        tunnel: w706 -> [w727 w732]
                        tunnel: [w727 w732] -> w705
                        tunnel: [w726 w731] -> w698
                        tunnel: w693 -> [w725 w730]
                        tunnel: [w725 w730] -> w692
                        tunnel: w688 -> [_ w729]
                        tunnel: [w724 w729] -> _
                        tunnel: w687 -> [w724 _]
                        frame "Channel_A_Rh1" {
                        }
                        frame "Channel_A_R", Default {
                        }
                      }
                      n146 = case shown="\"Channel_B_Rh1\"" "Channel B Waveform Display" {
                        tunnel: [w718 w721] -> w697
                        tunnel: w704 -> [w718 w723]
                        tunnel: [w718 w723] -> w703
                        tunnel: w702 -> [w717 w722]
                        tunnel: [w717 w722] -> w700
                        tunnel: [w716 w721] -> w701
                        tunnel: w699 -> [w716 w721]
                        tunnel: w694 -> [w715 w720]
                        tunnel: [w715 w720] -> w691
                        tunnel: w690 -> [_ w719]
                        tunnel: [w714 w719] -> _
                        tunnel: w689 -> [w714 _]
                        frame "Channel_B_R", Default {
                        }
                        frame "Channel_B_Rh1" {
                        }
                      }
                    }
                  }
                }
                n147 = call "OE1022D_Close.vi"("错误输入（无错误）"=w506, "VISA resource name"=w505) -> ("错误输出"=w504:errorcluster)  [unwired: 1 in]
              }
              frame #1 {
                n148 = Wait (ms)(milliseconds to wait=20) -> ()  [unwired: 1 out]
                "错误输出" <- w738
              }
              frame #2 {
                n149 = flat-sequence {
                  tunnel: w768 -> [w781]
                  tunnel: w769 -> [w782]
                  tunnel: w770 -> [w783]
                  tunnel: [w783] -> w774
                  tunnel: [w782] -> w773
                  tunnel: [w781] -> w772
                  tunnel: ["File Path"] -> w771
                  tunnel: [w778] -> w767
                  tunnel: w766 -> [w778]
                  tunnel: w765 -> [w777]
                  tunnel: [w777] -> w764
                  tunnel: w763 -> [w776]
                  tunnel: [w776] -> w762
                  tunnel: [w775] -> w760
                  tunnel: w759 -> [w775]
                  tunnel: w774 -> [w827]
                  tunnel: w773 -> [w830]
                  tunnel: w772 -> [w833]
                  tunnel: w771 -> [w840]
                  tunnel: w767 -> [w838]
                  tunnel: w764 -> [w837]
                  tunnel: w762 -> [w828]
                  tunnel: w761 -> [w829]
                  tunnel: w760 -> [w817]
                  tunnel: [w799] -> w758
                  tunnel: w757 -> [w815]
                  tunnel: w756 -> [w814]
                  tunnel: w755 -> [w811]
                  tunnel: w754 -> [w810]
                  tunnel: w753 -> [w804]
                  tunnel: w752 -> [w803]
                  tunnel: w751 -> [w799]
                  tunnel: w750 -> [w800]
                  tunnel: [w797] -> w749
                  tunnel: [w788] -> w748
                  tunnel: w747 -> [w798]
                  tunnel: w746 -> [w792]
                  tunnel: w745 -> [w790]
                  tunnel: w744 -> [w789]
                  tunnel: w743 -> [w786]
                  frame #0 {
                    n150 = case shown="True" FALSE {
                      tunnel: "File Path" -> [_ w785]
                      frame False {
                      }
                      frame True {
                        n151 = Write to Text File(file (use dialog)=w785, text="num_points Ra Rb\r\n") -> ()  [unwired: 2 in, 3 out]
                      }
                    }
                  }
                  frame #1 {
                    w820 = "stds"
                    w839 = TRUE
                    n152 = Add Array Elements(numeric array=w827) -> (sum=w844:dbl)
                    n153 = Add Array Elements(numeric array=w828) -> (sum=w835:dbl)
                    n154 = Add Array Elements(numeric array=w830) -> (sum=w842:dbl)
                    n155 = call <vilib>:"Std Deviation and Variance.vi"("X"=w830) -> ("mean"=w802:dbl, "standard deviation"=w821:dbl)  [unwired: 1 in, 1 out]
                    n156 = call <vilib>:"Std Deviation and Variance.vi"("X"=w828) -> ("mean"=w826:dbl, "standard deviation"=w823:dbl)  [unwired: 1 in, 1 out]
                    n157 = Divide(x=w844, y=w833) -> ()  [unwired: 1 out]
                    n158 = Divide(x=w835, y=w833) -> ()  [unwired: 1 out]
                    n159 = Divide(x=w842, y=w833) -> ()  [unwired: 1 out]
                    n160 = Add Array Elements(numeric array=w829) -> (sum=w834:dbl)
                    n161 = call <vilib>:"Std Deviation and Variance.vi"("X"=w827) -> ("mean"=w801:dbl, "standard deviation"=w822:dbl)  [unwired: 1 in, 1 out]
                    n162 = call <vilib>:"Std Deviation and Variance.vi"("X"=w829) -> ("mean"=w825:dbl, "standard deviation"=w824:dbl)  [unwired: 1 in, 1 out]
                    n163 = Divide(x=w834, y=w833) -> ()  [unwired: 1 out]
                    n164 = Build Array(w799, w790, w811, w810, w833, w801, w802, w826, w825, w822, w821, w823, w824, w804, w803, w815, w814) -> (w843:dbl[])
                    n165 = Equal To 0?(x=w817) -> (x = 0?=w816:bool)
                    n166 = Divide(x=w802, y=w801) -> (x/y=w794:dbl)
                    n167 = Build Array("Set Voltage 2450", "Actual Voltage 2450", "Set Voltage 2410", "Actual Voltage 2410", "NumPoints", w838, w837, "thetaA", "thetaB", w820, w820, w820, w820, "current25140 (uA)", "current2540Std (uA)", "current2410 (uA)", "current2410Std (uA)") -> (w836:string[])
                    n168 = Multiply(x=w794, y=100.0) -> (x*y=w795:dbl)
                    n169 = Build Array (concatenate)(w800, w795) -> (w797:dbl[])
                    n170 = case shown="True" w816 {
                      tunnel: [w846 w850] -> w841
                      tunnel: w840 -> [w846 w849]
                      tunnel: w839 -> [_ w848]
                      tunnel: w836 -> [_ w847]
                      frame False {
                      }
                      frame True {
                        n171 = call-poly <vilib>:"Write Delimited Spreadsheet.vi"("file path (dialog if empty)"=w849, "1D data"=w847, "append to file? (new file:F)"=w848) -> ("new file path (Not A Path if cancelled)"=w850:path)  [unwired: 11 in, 1 out]
                      }
                    }
                    n172 = Build Array (concatenate)(w798, w789) -> (w788:dbl[])
                    n173 = Bundle(w788, w792) -> (→"XY Graph 2":cluster{dbl[], dbl[]})  [unwired: 1 in]
                    n174 = Bundle(w788, w797) -> (→"XY Graph":cluster{dbl[], dbl[]})  [unwired: 1 in]
                    n175 = Bundle(w788, w786) -> (→"XY Graph 3":cluster{dbl[], dbl[]})  [unwired: 1 in]
                    n176 = call-poly <vilib>:"Write Delimited Spreadsheet.vi"("file path (dialog if empty)"=w841, "format (%.3f)"="%.10f", "1D data"=w843, "append to file? (new file:F)"=w839) -> ()  [unwired: 10 in, 2 out]
                  }
                }
              }
            }
          }
          frame #3 {
            n177 = Equal?(x=w852, y=w853) -> (x = y?=w851:bool)
            n178 = case shown="False" w851 {
              frame False {
              }
              frame True {
              }
            }
          }
        }
        n179 = Increment(x=w177) -> (x+1=w180:i32)
        n180 = Greater Or Equal?(x=w180, y=w146) -> (x >= y?=w181:bool)
        "Current set voltage 2450" <- w148
        "Current set voltage 2410" <- w147
        "current E field" <- w149
      }
    }
    frame True {
      n181 = case shown="True" w856 {
        tunnel: w855 -> [_ w866]
        frame False {
        }
        frame True {
          n182 = flat-sequence {
            tunnel: w866 -> [w880]
            frame #0 {
              w881 = TRUE  # Reset (True)
              n183 = call "Initialize.vi"("Serial Configuration"="Serial Configuration 2", "Reset (True)"=w881, "VISA resource name"=w880) -> ("error out"=w875:errorcluster, "VISA resource name out"=w876:refnum<visa-resource-name>)  [unwired: 7 in]
              n184 = call "Configure Measurement.vi"("error in (no error)"=w875, "VISA resource name"=w876) -> ("error out"=w867:errorcluster, "VISA resource name out"=w868:refnum<visa-resource-name>)  [unwired: 8 in]
              n185 = call "Configure Output.vi"("error in (no error)"=w867, "VISA resource name"=w868) -> ("error out"=w873:errorcluster, "VISA resource name out"=w874:refnum<visa-resource-name>)  [unwired: 8 in]
              n186 = call "Enable Output.vi"("error in (no error)"=w873, "VISA resource name"=w874) -> ("error out"=w871:errorcluster, "VISA resource name out"=w872:refnum<visa-resource-name>)  [unwired: 8 in]
              n187 = call-poly "Read.vi"("VISA resource name"=w872, "error in (no error)"=w871) -> ("VISA resource name out"=w869:refnum<visa-resource-name>, "error out"=w870:errorcluster)  [unwired: 7 in, 5 out]
              n188 = call "Enable Output.vi"("error in (no error)"=w870, "Enable Output (T: Enable)"=FALSE, "VISA resource name"=w869) -> ("error out"=w879:errorcluster, "VISA resource name out"=w878:refnum<visa-resource-name>)  [unwired: 7 in]
              n189 = call "Close.vi"("error in (no error)"=w879, "VISA resource name"=w878) -> ()  [unwired: 9 in, 1 out]
            }
            frame #1 {
              n190 = call "Display Message to User"() -> ()  [unwired: 10 in, 2 out]
            }
          }
        }
      }
      n191 = case shown="True" w857 {
        tunnel: w854 -> [_ w859]
        frame False {
        }
        frame True {
          w864 = TRUE  # Reset (True)
          w865 = TRUE  # ID Query (True)
          n192 = call "Initialize.vi"("Reset (True)"=w864, "ID Query (True)"=w865, "VISA resource name"=w859) -> ("error out"=w863:errorcluster, "VISA resource name out"=w862:refnum<visa-resource-name>)  [unwired: 7 in]
          n193 = call "Enable Output.vi"("error in (no error)"=w863, "Enable Output (T: Enable)"=FALSE, "VISA resource name"=w862) -> ("error out"=w860:errorcluster, "VISA resource name out"=w861:refnum<visa-resource-name>)  [unwired: 7 in]
          n194 = call "Close.vi"("error in (no error)"=w860, "VISA resource name"=w861) -> ()  [unwired: 9 in, 1 out]
        }
      }
    }
  }
